vi "PumpValve4.vi"() -> ()   [LabVIEW 2015]
uses:
  PumpValve.ctl
  <vilib>/DAQmx/write.llb/DAQmx Write (Digital 1D Bool NChan 1Samp 1Line).vi
  <vilib>/DAQmx/miscellaneous.llb/DAQmx Fill In Error Info.vi
panel:
  in  "On/Off (Pump)":bool
  in  "Open/Close (Blue)":bool
  in  "Open/Close (Green)":bool
  in  "Manual Mode":bool
  out "Invalid fill%":bool
  out "Tank":u32(slide) scale=0.0..100.0
  in  "Drain %":u32
  in  "Fill %":u32
  in  "Drain":bool
  in  "Stop Program":bool
  in  "Fill":bool
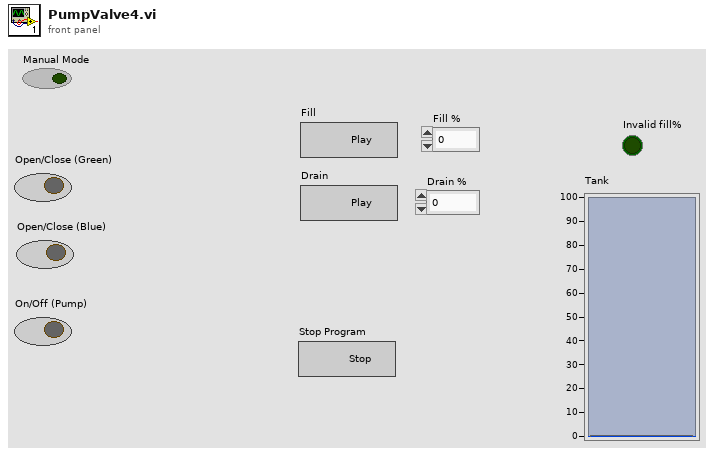
[diagram p1: front panel]
types:
  T1 = typedef "PumpValve.ctl" = enum16{"Manual", "Initialize", "Idle", "Fill", "Drain", "Stop"}
  T2 = cluster{"Open/Close (Green)":bool, "Open/Close (Blue)":bool, "On/Off (Pump)":bool}
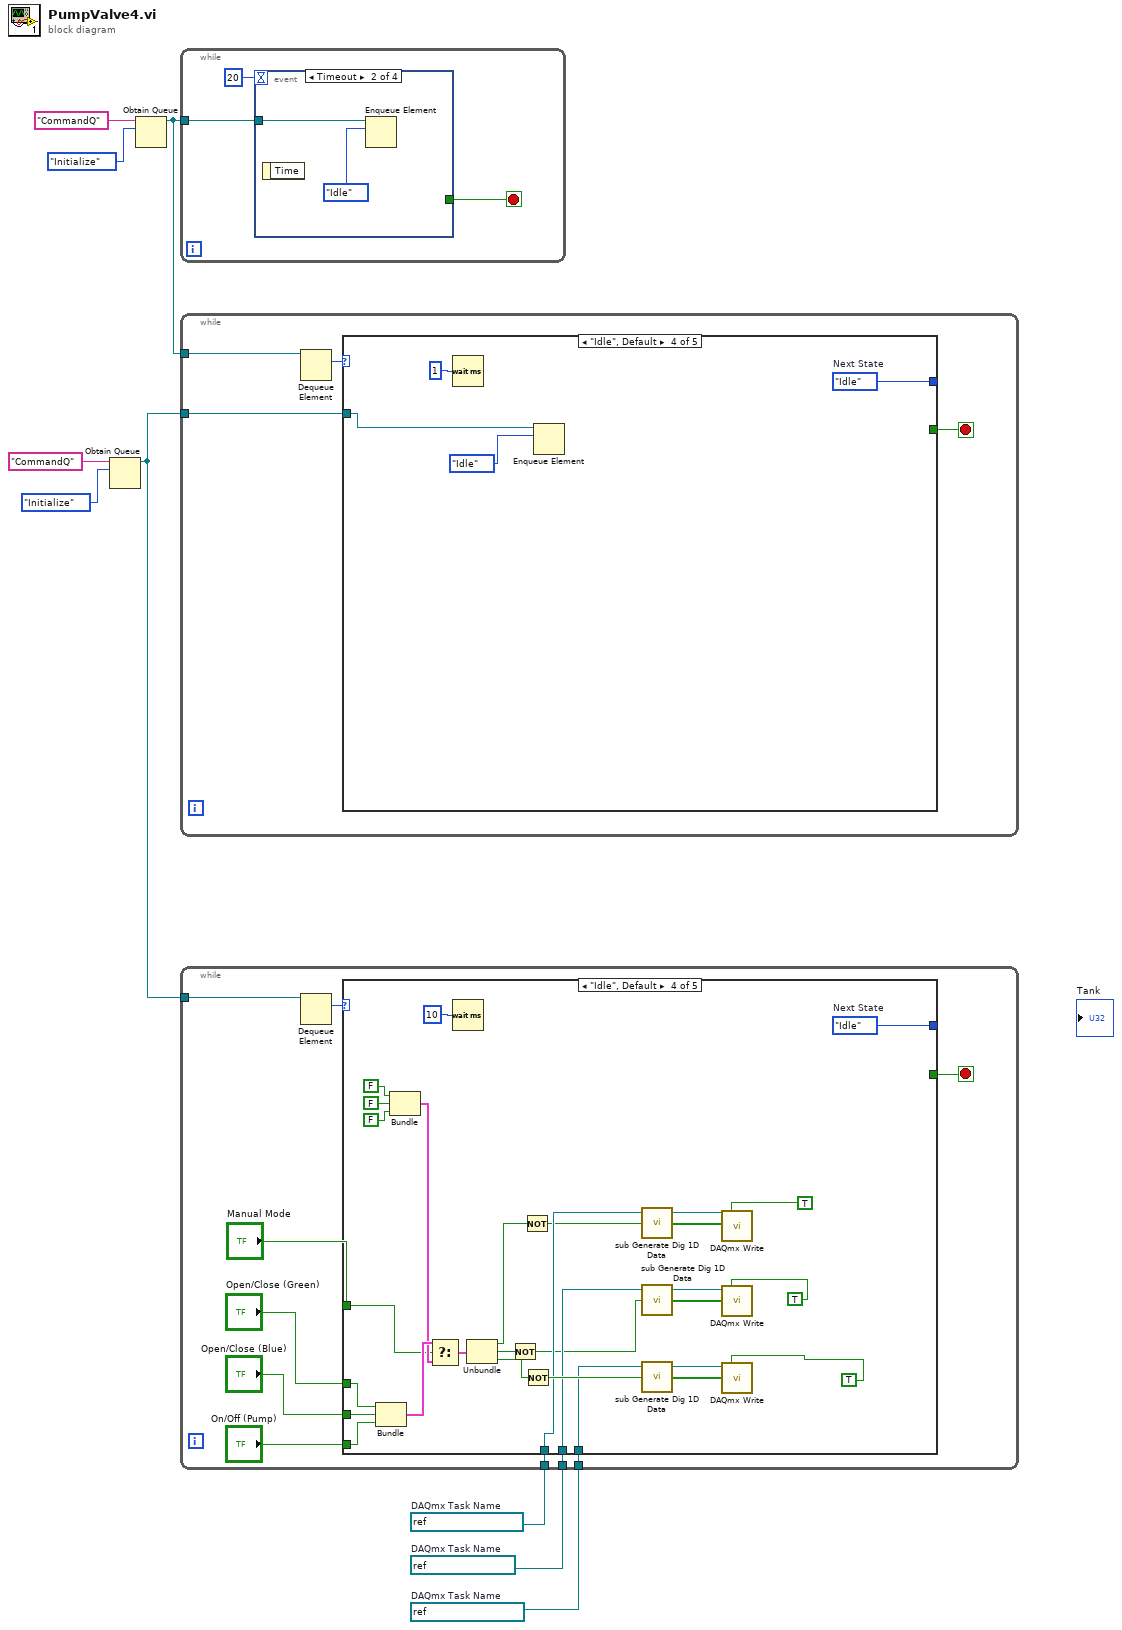
[diagram p0: block diagram]
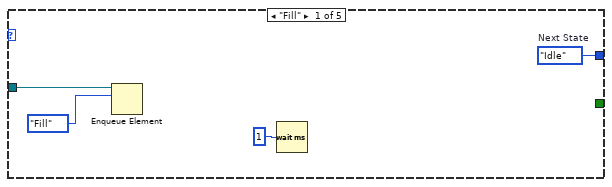
[diagram p2: hidden frame]
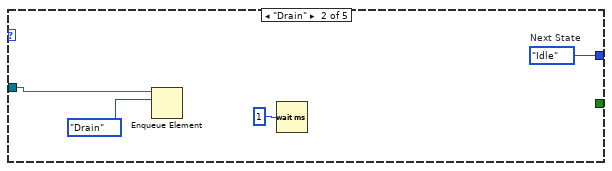
[diagram p3: hidden frame]
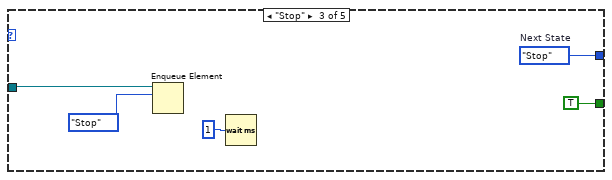
[diagram p4: hidden frame]
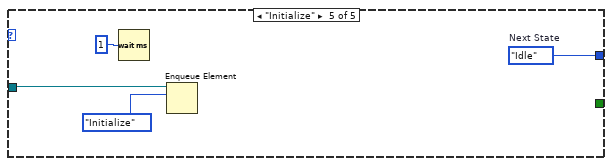
[diagram p5: hidden frame]
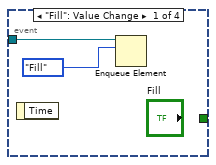
[diagram p6: hidden frame]
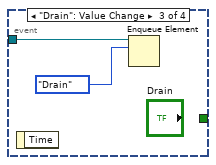
[diagram p7: hidden frame]
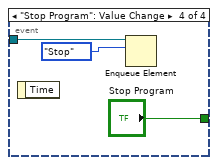
[diagram p8: hidden frame]
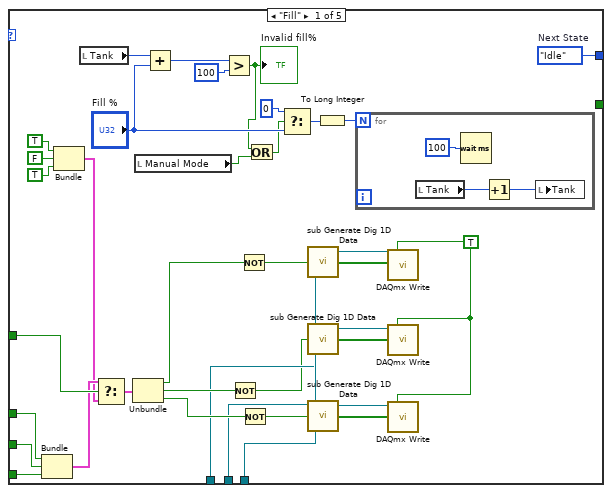
[diagram p9: hidden frame]
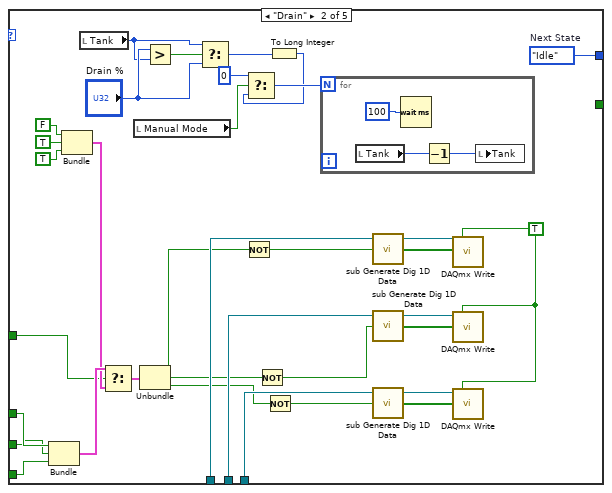
[diagram p10: hidden frame]
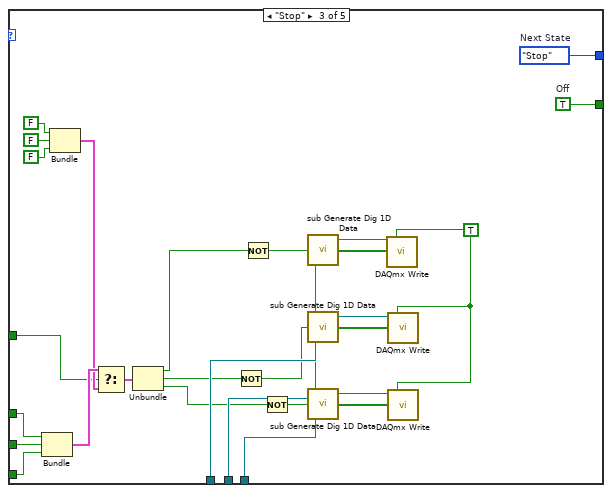
[diagram p11: hidden frame]
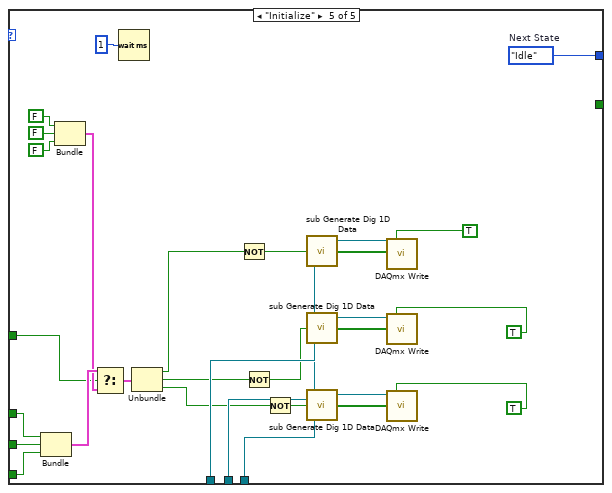
[diagram p12: hidden frame]
diagram:
  w5 = refnum<k21> "PumpTask-P0L0"  # DAQmx Task Name
  w6 = refnum<k21> "BlueTask-P0L1"  # DAQmx Task Name
  w7 = refnum<k21> "GreenTask-P0L2"  # DAQmx Task Name
  n1 = Obtain Queue(name (unnamed)="CommandQ", element data type=PumpValve."Initialize" ("States")) -> (queue out=w1:refnum<queue>)  [unwired: 3 in, 2 out]
  n2 = Obtain Queue(name (unnamed)="CommandQ", element data type=PumpValve."Initialize" ("States")) -> (queue out=w4:refnum<queue>)  [unwired: 3 in, 2 out]
  n3 = while {
    tunnel: w4 -> [w11]
    stop <- w10 stop-if-true
    n4 = event shown="[1] Timeout" {
      selector: _ -> [_ _ _ _]
      dyn-events: _ -> [_ _ _ _]
      timeout: 20 -> [_ _ _ _]
      tunnel: w11 -> [w14 w16 w18 w21]
      tunnel: [_ _ _ "Stop Program"] -> w10
      event "Fill": Value Change {
        n5 = event-data() -> ()  [unwired: 1 in, 1 out]
        n6 = Enqueue Element(queue=w14, element=PumpValve."Fill" ("States")) -> ()  [unwired: 2 in, 3 out]
      }
      event Timeout {
        n7 = event-data() -> ()  [unwired: 1 in, 1 out]
        n8 = Enqueue Element(queue=w16, element=PumpValve."Idle" ("States")) -> ()  [unwired: 2 in, 3 out]
      }
      event "Drain": Value Change {
        n9 = event-data() -> ()  [unwired: 1 in, 1 out]
        n10 = Enqueue Element(queue=w18, element=PumpValve."Drain" ("States")) -> ()  [unwired: 2 in, 3 out]
      }
      event "Stop Program": Value Change {
        n11 = event-data() -> ()  [unwired: 1 in, 1 out]
        n12 = Enqueue Element(queue=w21, element=PumpValve."Stop" ("States")) -> ()  [unwired: 2 in, 3 out]
      }
    }
  }
  n13 = while {
    tunnel: w4 -> [w24]
    tunnel: w1 -> [w23]
    stop <- w22 stop-if-true
    n14 = Dequeue Element(queue=w24) -> (element=w25:T1)  [unwired: 2 in, 3 out]
    n15 = case shown="\"Idle\", Default" w25 {
      tunnel: [w29 w33 w38 w42 w46] -> _
      tunnel: w23 -> [w26 w30 w35 w39 w43]
      tunnel: [_ _ TRUE _ _] -> w22
      frame "Fill" {
        w29 = PumpValve."Idle"  # Next State
        n16 = Enqueue Element(queue=w26, element=PumpValve."Fill" ("States")) -> ()  [unwired: 2 in, 3 out]
        n17 = Wait (ms)(milliseconds to wait=u32 1) -> ()  [unwired: 1 out]
      }
      frame "Drain" {
        w33 = PumpValve."Idle"  # Next State
        n18 = Enqueue Element(queue=w30, element=PumpValve."Drain" ("States")) -> ()  [unwired: 2 in, 3 out]
        n19 = Wait (ms)(milliseconds to wait=u32 1) -> ()  [unwired: 1 out]
      }
      frame "Stop" {
        w38 = PumpValve."Stop"  # Next State
        n20 = Enqueue Element(queue=w35, element=PumpValve."Stop" ("States")) -> ()  [unwired: 2 in, 3 out]
        n21 = Wait (ms)(milliseconds to wait=u32 1) -> ()  [unwired: 1 out]
      }
      frame "Idle", Default {
        w42 = PumpValve."Idle"  # Next State
        n22 = Wait (ms)(milliseconds to wait=u32 1) -> ()  [unwired: 1 out]
        n23 = Enqueue Element(queue=w39, element=PumpValve."Idle" ("States")) -> ()  [unwired: 2 in, 3 out]
      }
      frame "Initialize" {
        w46 = PumpValve."Idle"  # Next State
        n24 = Wait (ms)(milliseconds to wait=u32 1) -> ()  [unwired: 1 out]
        n25 = Enqueue Element(queue=w43, element=PumpValve."Initialize" ("States")) -> ()  [unwired: 2 in, 3 out]
      }
    }
  }
  n26 = while {
    tunnel: w1 -> [w56]
    tunnel: w7 -> [w47]
    tunnel: w6 -> [w48]
    tunnel: w5 -> [w49]
    stop <- w55 stop-if-true
    n27 = Dequeue Element(queue=w56) -> (element=w54:T1)  [unwired: 2 in, 3 out]
    n28 = case shown="\"Idle\", Default" w54 {
      tunnel: [w93 w131 w162 w192 w222] -> _
      tunnel: [_ _ w135 _ _] -> w55
      tunnel: "Open/Close (Blue)" -> [w79 w107 w143 w175 w202]
      tunnel: "Open/Close (Green)" -> [w78 w108 w144 w176 w203]
      tunnel: "On/Off (Pump)" -> [w77 w106 w142 w174 w201]
      tunnel: "Manual Mode" -> [w76 w109 w145 w177 w204]
      tunnel: w49 -> [w62 w103 w147 w167 w206]
      tunnel: w48 -> [w61 w104 w148 w166 w207]
      tunnel: w47 -> [w60 w105 w149 w165 w208]
      frame "Fill" {
        w72 = TRUE
        w93 = PumpValve."Idle"  # Next State
        n29 = Bundle("Open/Close (Green)"=w78, "Open/Close (Blue)"=w79, "On/Off (Pump)"=w77) -> (w75:T2)  [unwired: 1 in]
        n30 = Bundle(TRUE, FALSE, TRUE) -> (w74:cluster{bool, bool, bool})  [unwired: 1 in]
        n31 = local read "Tank"() -> (w92:u32)
        n32 = Select(t=w75, s=w76, f=w74) -> (s? t:f=w73:T2)
        n33 = Unbundle(w73) -> ("Open/Close (Green)"=w65:bool, "Open/Close (Blue)"=w64:bool, "On/Off (Pump)"=w63:bool)
        n34 = local read "Manual Mode"() -> (w81:bool)
        n35 = Add(x=w92, y="Fill %") -> (x+y=w90:u32)
        n36 = Greater?(x=w90, y=u32 100) -> (0:w82:bool)
        "Invalid fill%" <- w82
        n37 = Not(x=w64) -> (.not. x?=w57:bool)
        n38 = Not(x=w65) -> (.not. x?=w58:bool)
        n39 = Not(x=w63) -> (.not. x?=w59:bool)
        n40 = Or(x=w82, y=w81) -> (x .or. y?=w80:bool)
        n41 = Select(t=u32 0, s=w80, f="Fill %") -> (s? t:f=w87:u32)
        n42 = call <vilib>:"sub Generate Dig 1D Data.vi"("initial value"=w58, "task in"=w60) -> ("Data"=w67:bool[], "task out"=w71:refnum<k21>)  [unwired: 1 in, 1 out]
        n43 = call <vilib>:"sub Generate Dig 1D Data.vi"("initial value"=w57, "task in"=w61) -> ("Data"=w68:bool[], "task out"=w70:refnum<k21>)  [unwired: 1 in, 1 out]
        n44 = call <vilib>:"sub Generate Dig 1D Data.vi"("initial value"=w59, "task in"=w62) -> ("Data"=w66:bool[], "task out"=w69:refnum<k21>)  [unwired: 1 in, 1 out]
        n45 = To Long Integer(number=w87) -> (32bit integer=w86:i32)
        n46 = for {
          N: w86 -> [_]
          n47 = local read "Tank"() -> (w96:u32)
          n48 = Wait (ms)(milliseconds to wait=u32 100 ("y")) -> ()  [unwired: 1 out]
          n49 = Increment(x=w96) -> (x+1=w95:u32)
          n50 = local write "Tank"(w95) -> ()
        }
        n51 = call-poly <vilib>:"DAQmx Write.vi"("task/channels in"=w71, "auto start"=w72, "data"=w67) -> ()  [unwired: 10 in, 3 out]
        n52 = call-poly <vilib>:"DAQmx Write.vi"("task/channels in"=w70, "auto start"=w72, "data"=w68) -> ()  [unwired: 10 in, 3 out]
        n53 = call-poly <vilib>:"DAQmx Write.vi"("task/channels in"=w69, "auto start"=w72, "data"=w66) -> ()  [unwired: 10 in, 3 out]
      }
      frame "Drain" {
        w113 = TRUE
        w131 = PumpValve."Idle"  # Next State
        n54 = Bundle("Open/Close (Green)"=w108, "Open/Close (Blue)"=w107, "On/Off (Pump)"=w106) -> (w111:T2)  [unwired: 1 in]
        n55 = Bundle(FALSE, TRUE, TRUE) -> (w110:cluster{bool, bool, bool})  [unwired: 1 in]
        n56 = local read "Tank"() -> (w128:u32)
        n57 = Select(t=w111, s=w109, f=w110) -> (s? t:f=w112:T2)
        n58 = local read "Manual Mode"() -> (w123:bool)
        n59 = Unbundle(w112) -> ("Open/Close (Green)"=w102:bool, "Open/Close (Blue)"=w101:bool, "On/Off (Pump)"=w100:bool)
        n60 = Greater?(x="Drain %", y=w128) -> (0:w124:bool)
        n61 = Select(t=w128, s=w124, f="Drain %") -> (s? t:f=w130:u32)
        n62 = Not(x=w102) -> (.not. x?=w98:bool)
        n63 = Not(x=w101) -> (.not. x?=w97:bool)
        n64 = Not(x=w100) -> (.not. x?=w99:bool)
        n65 = To Long Integer(number=w130) -> (32bit integer=w120:i32)
        n66 = Select(t=0, s=w123, f=w120) -> (s? t:f=w121:i32)
        n67 = for {
          N: w121 -> [_]
          n68 = local read "Tank"() -> (w133:u32)
          n69 = Wait (ms)(milliseconds to wait=u32 100) -> ()  [unwired: 1 out]
          n70 = Decrement(x=w133) -> (x-1=w134:u32)
          n71 = local write "Tank"(w134) -> ()
        }
        n72 = call <vilib>:"sub Generate Dig 1D Data.vi"("initial value"=w98, "task in"=w105) -> ("Data"=w118:bool[], "task out"=w114:refnum<k21>)  [unwired: 1 in, 1 out]
        n73 = call <vilib>:"sub Generate Dig 1D Data.vi"("initial value"=w97, "task in"=w104) -> ("Data"=w117:bool[], "task out"=w115:refnum<k21>)  [unwired: 1 in, 1 out]
        n74 = call <vilib>:"sub Generate Dig 1D Data.vi"("initial value"=w99, "task in"=w103) -> ("Data"=w119:bool[], "task out"=w116:refnum<k21>)  [unwired: 1 in, 1 out]
        n75 = call-poly <vilib>:"DAQmx Write.vi"("task/channels in"=w114, "auto start"=w113, "data"=w118) -> ()  [unwired: 10 in, 3 out]
        n76 = call-poly <vilib>:"DAQmx Write.vi"("task/channels in"=w115, "auto start"=w113, "data"=w117) -> ()  [unwired: 10 in, 3 out]
        n77 = call-poly <vilib>:"DAQmx Write.vi"("task/channels in"=w116, "auto start"=w113, "data"=w119) -> ()  [unwired: 10 in, 3 out]
      }
      frame "Stop" {
        w156 = TRUE
        w135 = TRUE  # Off
        w162 = PumpValve."Stop"  # Next State
        n78 = Bundle("Open/Close (Green)"=w144, "Open/Close (Blue)"=w143, "On/Off (Pump)"=w142) -> (w158:T2)  [unwired: 1 in]
        n79 = Bundle(FALSE, FALSE, FALSE) -> (w146:cluster{bool, bool, bool})  [unwired: 1 in]
        n80 = Select(t=w158, s=w145, f=w146) -> (s? t:f=w157:T2)
        n81 = Unbundle(w157) -> ("Open/Close (Green)"=w141:bool, "Open/Close (Blue)"=w140:bool, "On/Off (Pump)"=w139:bool)
        n82 = Not(x=w140) -> (.not. x?=w136:bool)
        n83 = Not(x=w141) -> (.not. x?=w137:bool)
        n84 = Not(x=w139) -> (.not. x?=w138:bool)
        n85 = call <vilib>:"sub Generate Dig 1D Data.vi"("initial value"=w137, "task in"=w149) -> ("Data"=w151:bool[], "task out"=w155:refnum<k21>)  [unwired: 1 in, 1 out]
        n86 = call <vilib>:"sub Generate Dig 1D Data.vi"("initial value"=w136, "task in"=w148) -> ("Data"=w152:bool[], "task out"=w154:refnum<k21>)  [unwired: 1 in, 1 out]
        n87 = call <vilib>:"sub Generate Dig 1D Data.vi"("initial value"=w138, "task in"=w147) -> ("Data"=w150:bool[], "task out"=w153:refnum<k21>)  [unwired: 1 in, 1 out]
        n88 = call-poly <vilib>:"DAQmx Write.vi"("task/channels in"=w155, "auto start"=w156, "data"=w151) -> ()  [unwired: 10 in, 3 out]
        n89 = call-poly <vilib>:"DAQmx Write.vi"("task/channels in"=w154, "auto start"=w156, "data"=w152) -> ()  [unwired: 10 in, 3 out]
        n90 = call-poly <vilib>:"DAQmx Write.vi"("task/channels in"=w153, "auto start"=w156, "data"=w150) -> ()  [unwired: 10 in, 3 out]
      }
      frame "Idle", Default {
        w192 = PumpValve."Idle"  # Next State
        n91 = Bundle("Open/Close (Green)"=w176, "Open/Close (Blue)"=w175, "On/Off (Pump)"=w174) -> (w187:T2)  [unwired: 1 in]
        n92 = Bundle(FALSE, FALSE, FALSE) -> (w178:cluster{bool, bool, bool})  [unwired: 1 in]
        n93 = Select(t=w187, s=w177, f=w178) -> (s? t:f=w186:T2)
        n94 = Wait (ms)(milliseconds to wait=u32 10) -> ()  [unwired: 1 out]
        n95 = Unbundle(w186) -> ("Open/Close (Green)"=w173:bool, "Open/Close (Blue)"=w172:bool, "On/Off (Pump)"=w171:bool)
        n96 = Not(x=w172) -> (.not. x?=w163:bool)
        n97 = Not(x=w173) -> (.not. x?=w164:bool)
        n98 = Not(x=w171) -> (.not. x?=w170:bool)
        n99 = call <vilib>:"sub Generate Dig 1D Data.vi"("initial value"=w164, "task in"=w165) -> ("Data"=w180:bool[], "task out"=w184:refnum<k21>)  [unwired: 1 in, 1 out]
        n100 = call <vilib>:"sub Generate Dig 1D Data.vi"("initial value"=w163, "task in"=w166) -> ("Data"=w181:bool[], "task out"=w183:refnum<k21>)  [unwired: 1 in, 1 out]
        n101 = call <vilib>:"sub Generate Dig 1D Data.vi"("initial value"=w170, "task in"=w167) -> ("Data"=w179:bool[], "task out"=w182:refnum<k21>)  [unwired: 1 in, 1 out]
        n102 = call-poly <vilib>:"DAQmx Write.vi"("task/channels in"=w184, "auto start"=TRUE, "data"=w180) -> ()  [unwired: 10 in, 3 out]
        n103 = call-poly <vilib>:"DAQmx Write.vi"("task/channels in"=w183, "auto start"=TRUE, "data"=w181) -> ()  [unwired: 10 in, 3 out]
        n104 = call-poly <vilib>:"DAQmx Write.vi"("task/channels in"=w182, "auto start"=TRUE, "data"=w179) -> ()  [unwired: 10 in, 3 out]
      }
      frame "Initialize" {
        w222 = PumpValve."Idle"  # Next State
        n105 = Bundle("Open/Close (Green)"=w203, "Open/Close (Blue)"=w202, "On/Off (Pump)"=w201) -> (w217:T2)  [unwired: 1 in]
        n106 = Bundle(FALSE, FALSE, FALSE) -> (w205:cluster{bool, bool, bool})  [unwired: 1 in]
        n107 = Select(t=w217, s=w204, f=w205) -> (s? t:f=w216:T2)
        n108 = Wait (ms)(milliseconds to wait=u32 1) -> ()  [unwired: 1 out]
        n109 = Unbundle(w216) -> ("Open/Close (Green)"=w200:bool, "Open/Close (Blue)"=w199:bool, "On/Off (Pump)"=w198:bool)
        n110 = Not(x=w200) -> (.not. x?=w194:bool)
        n111 = Not(x=w199) -> (.not. x?=w193:bool)
        n112 = Not(x=w198) -> (.not. x?=w197:bool)
        n113 = call <vilib>:"sub Generate Dig 1D Data.vi"("initial value"=w194, "task in"=w208) -> ("Data"=w210:bool[], "task out"=w214:refnum<k21>)  [unwired: 1 in, 1 out]
        n114 = call <vilib>:"sub Generate Dig 1D Data.vi"("initial value"=w193, "task in"=w207) -> ("Data"=w211:bool[], "task out"=w213:refnum<k21>)  [unwired: 1 in, 1 out]
        n115 = call <vilib>:"sub Generate Dig 1D Data.vi"("initial value"=w197, "task in"=w206) -> ("Data"=w209:bool[], "task out"=w212:refnum<k21>)  [unwired: 1 in, 1 out]
        n116 = call-poly <vilib>:"DAQmx Write.vi"("task/channels in"=w214, "auto start"=TRUE, "data"=w210) -> ()  [unwired: 10 in, 3 out]
        n117 = call-poly <vilib>:"DAQmx Write.vi"("task/channels in"=w213, "auto start"=TRUE, "data"=w211) -> ()  [unwired: 10 in, 3 out]
        n118 = call-poly <vilib>:"DAQmx Write.vi"("task/channels in"=w212, "auto start"=TRUE, "data"=w209) -> ()  [unwired: 10 in, 3 out]
      }
    }
  }
